vi "_Highlight Item.vi"(8 "error in":errorcluster, 10 "Item Tag":string) -> (0 "error out":errorcluster)   [LabVIEW 2020, in "Panther Dasboard Scripting Hooks.lvlib"]
uses:
  Panther Dasboard Scripting Hooks.lvlib
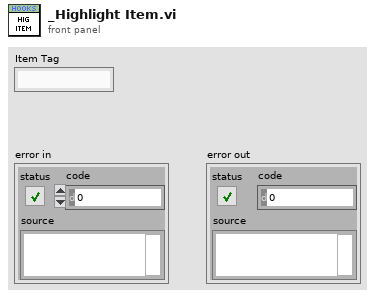
[diagram p1: front panel]
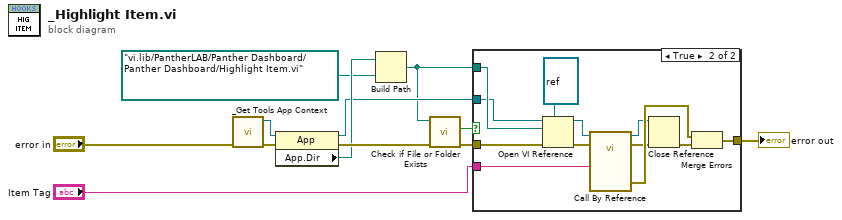
[diagram p0: block diagram]
diagram:
  n1 = call "_Get Tools App Context.vi"("error in"="error in") -> ("error out"=w10:errorcluster, "Application Context"=w5:refnum<vi>)  [unwired: 9 in]
  n2 = property class="App"(reference=w5, error in=w10) -> (reference out=w4:refnum<vi>, error out=w11:errorcluster, "App.Dir"=w7:path)
  n3 = Build Path(base path=w7, name or relative path=path "vi.lib/PantherLAB/Panther Dashboard/Panther Dashboard/Highlight Item.vi") -> (appended path=w2:path)
  n4 = call <vilib>:"Check if File or Folder Exists.vi"("error in (no error)"=w11, "path"=w2) -> ("error out"=w8:errorcluster, "file or folder exists?"=w1:bool)  [unwired: 7 in, 1 out]
  n5 = case shown="True" w1 {
    tunnel: [w13 w24] -> w12
    tunnel: w8 -> [w13 w22]
    tunnel: w2 -> [_ w18]
    tunnel: w4 -> [_ w15]
    tunnel: "Item Tag" -> [_ w14]
    frame False {
    }
    frame True {
      n6 = Open VI Reference(type specifier VI Refnum (for type only)=refnum<vi> refnum, application reference (local)=w15, vi path=w18, error in (no error)=w22) -> (vi reference=w17:refnum<vi>, error out=w21:errorcluster)  [unwired: 2 in]
      n7 = call-by-ref "?"(reference=w17, error in=w21, "Item Tag"=w14) -> (reference out=w16:refnum<vi>, error out=w20:errorcluster, 0:"error out"=w25:errorcluster)  [unwired: 10 in]
      n8 = Close Reference(reference=w16, error in (no error)=w20) -> (error out=w23:errorcluster)
      n9 = Merge Errors(w25, w23) -> (w24:errorcluster)
    }
  }
  "error out" <- w12
